vi "svc_Convert Spectrum Array to dB.vi"(9 "dB reference":dbl=1.0 format="%0.2f", 10 "spectrum type":T1=enum."Power [Magnitude^2]", 11 "spectrum":dbl[](array[numeric]) format="%0.2f") -> (3 "spectrum in dB":dbl[](array[numeric]) format="%0.2f")   [LabVIEW 2017]
uses:
  <vilib>/addons/_NISVFA/_Shared subVIs/Controls/svc_Spectrum Type.ctl
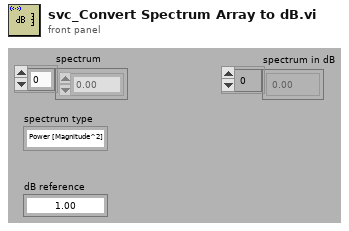
[diagram p1: front panel]
types:
  T1 = typedef "svc_Spectrum Type.ctl" = enum16{"FFT Spectrum [complex]", "Amplitude [Magnitude]", "Power [Magnitude^2]", "Cross Spectrum [complex]", "Frequency Response [Complex]"}
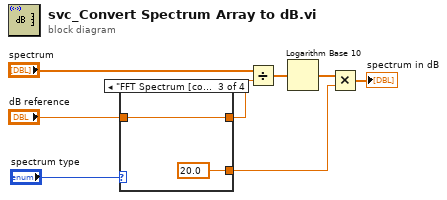
[diagram p0: block diagram]
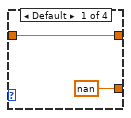
[diagram p2: hidden frame]
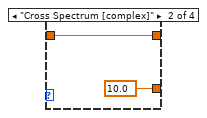
[diagram p3: hidden frame]
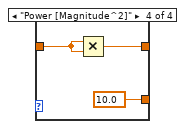
[diagram p4: hidden frame]
diagram:
  n1 = case shown="\"FFT Spectrum [complex]\", \"Amplitude [Magnitude]\", \"Frequency Response [Complex]\"" "spectrum type" {
    tunnel: "dB reference" -> [w10 w11 w14 w16]
    tunnel: [w10 w11 w14 w17] -> w3
    tunnel: [nan ("y") 10.0 ("y") 20.0 ("y") 10.0 ("y")] -> w1
    frame Default {
    }
    frame "Cross Spectrum [complex]" {
    }
    frame "FFT Spectrum [complex]", "Amplitude [Magnitude]", "Frequency Response [Complex]" {
    }
    frame "Power [Magnitude^2]" {
      n2 = Multiply(x=w16, y=w16) -> (x*y=w17:dbl)
    }
  }
  n3 = Divide(x="spectrum", y=w3) -> (x/y=w8:dbl[])
  n4 = Logarithm Base 10(1:w8) -> (0:w7:dbl[])
  n5 = Multiply(x=w7, y=w1) -> (x*y=→"spectrum in dB":dbl[])
